vi "Load States.vi"(8 "Error In":errorcluster, 10 "States Nodes":refnum<k20>[](array[refnum]), 11 "UIPs":string[](array[string])) -> (0 "Error Out":errorcluster, 3 "States Variant":variant)   [LabVIEW 2015, in "UIM.lvclass"]
uses:
  UIM.lvclass
  UIP/UIP.lvclass
  <vilib>/xml/Close Reference(Node).vi
  <resource>/objmgr/DOMUserDefRef.rc
  <vilib>/xml/NI_XML.lvlib
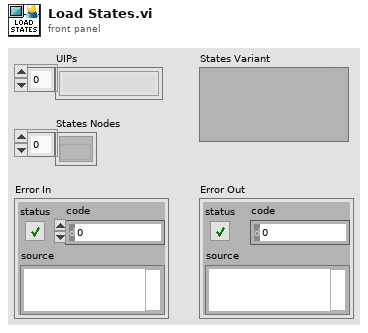
[diagram p1: front panel]
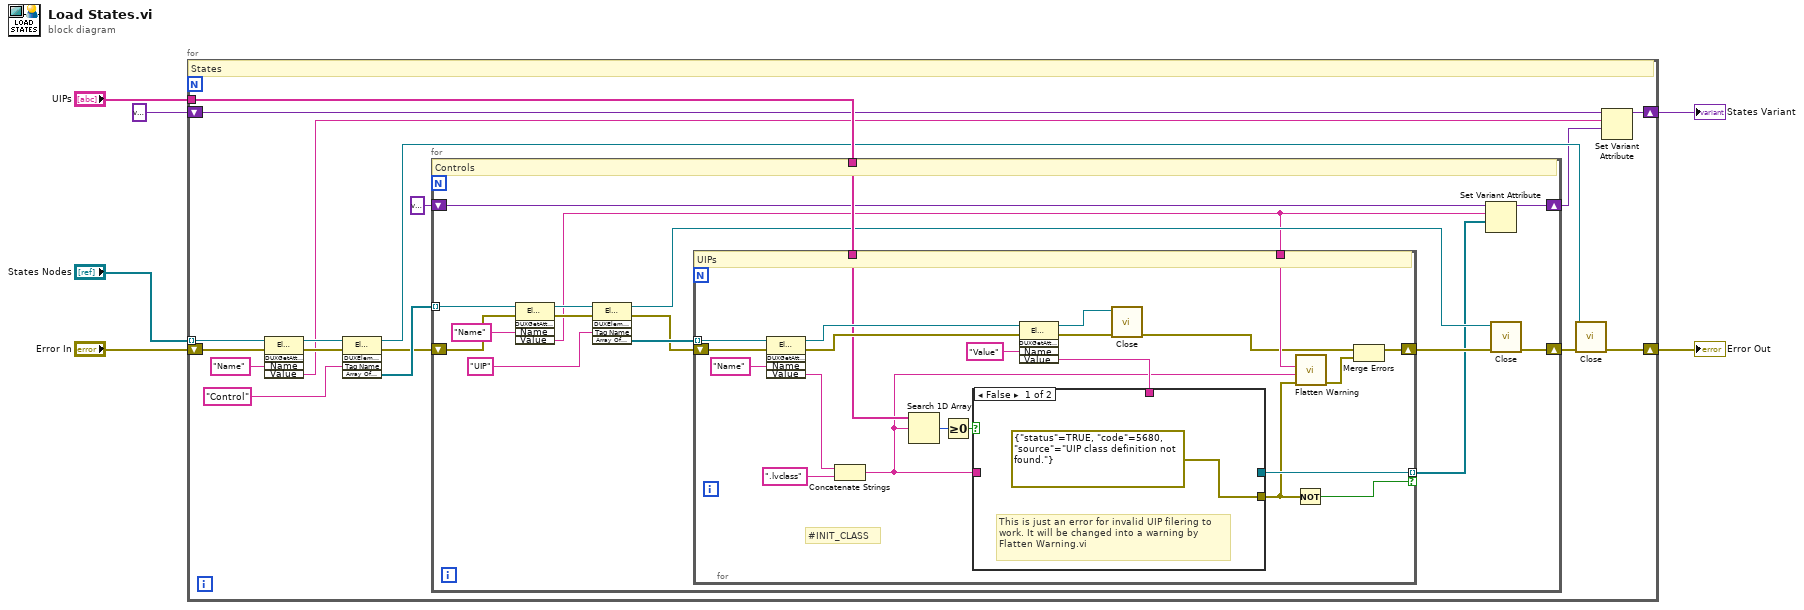
[diagram p0: block diagram]
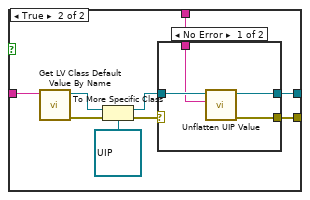
[diagram p2: hidden frame]
diagram:
  n1 = for {
    tunnel: "States Nodes" -> [w23] mode=indexing
    shift-right: [w9] -> w2
    shift-left: variant -> [w10]
    shift-right: [w14] -> w3
    shift-left: "Error In" -> [w18]
    tunnel: "UIPs" -> [w17]
    # "States"
    n2 = invoke class="Element" method="DUXGetAttribute"(reference=w23, error in=w18, "Name"="Name") -> (reference out=w21:refnum<k20>, error out=w13:errorcluster, "Value"=w7:string)  [unwired: 2 in, 2 out]
    n3 = invoke class="Element" method="DUXElementGetElementsByTagNameArray"(reference=w21, error in=w13, "Tag Name"="Control") -> (reference out=w15:refnum<k20>, error out=w12:errorcluster, "Array Of Elements"=w19:refnum<k20>[])  [unwired: 2 in, 2 out]
    n4 = for {
      tunnel: w19 -> [w39] mode=indexing
      shift-right: [w30] -> w16
      shift-left: w12 -> [w34]
      tunnel: w17 -> [w31]
      shift-right: [w24] -> w8
      shift-left: variant -> [w27]
      # "Controls"
      n5 = invoke class="Element" method="DUXGetAttribute"(reference=w39, error in=w34, "Name"="Name") -> (reference out=w37:refnum<k20>, error out=w33:errorcluster, "Value"=w26:string)  [unwired: 2 in, 2 out]
      n6 = invoke class="Element" method="DUXElementGetElementsByTagNameArray"(reference=w37, error in=w33, "Tag Name"="UIP") -> (reference out=w29:refnum<k20>, error out=w32:errorcluster, "Array Of Elements"=w35:refnum<k20>[])  [unwired: 2 in, 2 out]
      n7 = for {
        tunnel: w35 -> [w61] mode=indexing
        tunnel: w26 -> [w53]
        tunnel: [w51] -> w25 mode=indexing if=w49
        shift-right: [w48] -> w28
        shift-left: w32 -> [w57]
        tunnel: w31 -> [w41]
        # "#INIT_CLASS"
        # "UIPs"
        n8 = invoke class="Element" method="DUXGetAttribute"(reference=w61, error in=w57, "Name"="Name") -> (reference out=w60:refnum<k20>, error out=w56:errorcluster, "Value"=w52:string)  [unwired: 2 in, 2 out]
        n9 = Concatenate Strings(w52, ".lvclass" ("string")) -> (w40:string)
        n10 = Search 1D Array(1D array=w41, element=w40) -> (index of element=w43:i32)  [unwired: 1 in]
        n11 = Greater Or Equal To 0?(x=w43) -> (x >= 0?=w42:bool)
        n12 = invoke class="Element" method="DUXGetAttribute"(reference=w60, error in=w56, "Name"="Value") -> (reference out=w45:refnum<k20>, error out=w46:errorcluster, "Value"=w54:string)  [unwired: 2 in, 2 out]
        n13 = case shown="False" w42 {
          tunnel: w54 -> [_ w66]
          tunnel: [_ w65] -> w51
          tunnel: [errorcluster {"status"=TRUE, "code"=5680, "source"="UIP class definition not found."} ("error constant") w64] -> w50
          tunnel: w40 -> [_ w63]
          frame False {
            # "This is just an error for invalid UIP filering to\nwork. It will be changed into a warning by\nFlatten Warning.vi"
          }
          frame True {
            n14 = call <vilib>:"Get LV Class Default Value By Name.vi"("class name"=w63) -> ("error out"=w70:errorcluster, "object"=w71:refnum<class>)  [unwired: 9 in]
            n15 = To More Specific Class(target class=refnum<class "UIP.lvclass"> refnum ("UIP.lvclass"), reference=w71, error in=w70) -> (specific class reference=w67:refnum<class "UIP.lvclass">, error out=w68:errorcluster)
            n16 = case shown="No Error" w68 {
              selector: w68 -> [_ w76]
              tunnel: w67 -> [w75 _]
              tunnel: w66 -> [w74 _]
              tunnel: [w73 w76] -> w64
              tunnel: [w72 _] -> w65
              frame No Error {
                n17 = call-dynamic "Unflatten UIP Value.vi"("String Value"=w74, "UIP In"=w75) -> ("Error Out"=w73:errorcluster, "UIP Out"=w72:refnum<class "UIP.lvclass">)  [unwired: 8 in]
              }
              frame Error {
              }
            }
          }
        }
        n18 = call-poly <vilib>:"Close.vi"("error in (no error)"=w46, "node"=w45) -> ("error out"=w44:errorcluster)  [unwired: 7 in]
        n19 = Not(x=w50) -> (.not. x?=w49:bool)
        n20 = call "Flatten Warning.vi"("Error In"=w50, "UIP Name"=w40, "Label.Text"=w53) -> ("Error Out"=w47:errorcluster)  [unwired: 8 in]
        n21 = Merge Errors(w44, w47) -> (w48:errorcluster)
      }
      n22 = Set Variant Attribute(Variant=w27, name=w26, value=w25) -> (Variant out=w24:variant)  [unwired: 1 in, 2 out]
      n23 = call-poly <vilib>:"Close.vi"("error in (no error)"=w28, "node"=w29) -> ("error out"=w30:errorcluster)  [unwired: 7 in]
    }
    n24 = call-poly <vilib>:"Close.vi"("error in (no error)"=w16, "node"=w15) -> ("error out"=w14:errorcluster)  [unwired: 7 in]
    n25 = Set Variant Attribute(Variant=w10, name=w7, value=w8) -> (Variant out=w9:variant)  [unwired: 1 in, 2 out]
  }
  "Error Out" <- w3
  "States Variant" <- w2
